vi "GetControlValues.vi"(11 "VI Name":string) -> (3 "Values":string[](array[string]))   [LabVIEW 2018, in "TracerLibrary.lvlib" / "Tracer.lvclass"]
uses:
  Tracer.lvclass
  Tracer_ClassAttributes.vi
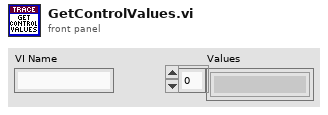
[diagram p1: front panel]
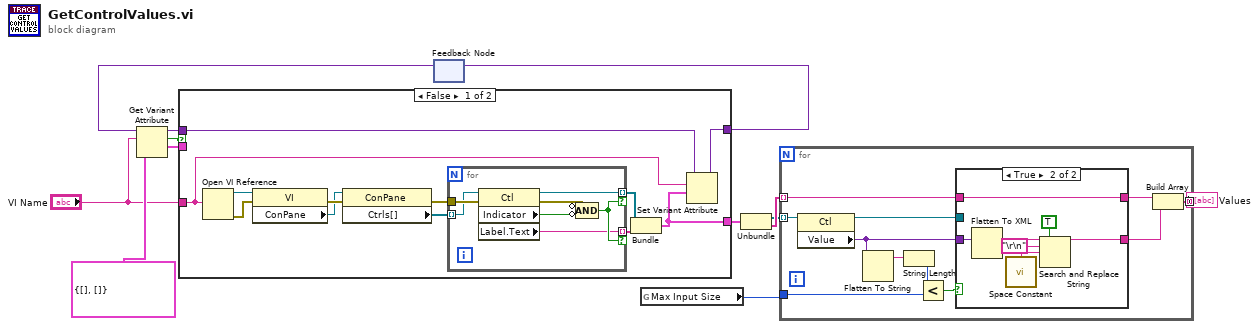
[diagram p0: block diagram]
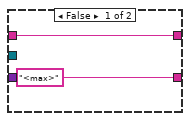
[diagram p2: hidden frame]
diagram:
  n1 = feedback #1() -> (w12:variant)  [unwired: 1 in]
  n2 = Get Variant Attribute(Variant=w12, name="VI Name", default value (empty Variant)=cluster{refnum<vi>[], string[]} {[], []} ("output cluster")) -> (duplicate Variant=w3:variant, found=w4:bool, value=w5:cluster{refnum<vi>[], string[]})  [unwired: 1 in, 1 out]
  n3 = case shown="False" w4 {
    tunnel: "VI Name" -> [w13 _]
    tunnel: w3 -> [w18 w32]
    tunnel: [w17 w32] -> w11
    tunnel: [w14 w33] -> w7
    tunnel: w5 -> [_ w33]
    frame False {
      n4 = Open VI Reference(vi path=w13) -> (vi reference=w21:refnum<vi>, error out=w23:errorcluster)  [unwired: 5 in]
      n5 = property class="VI"(reference=w21, error in=w23) -> (error out=w22:errorcluster, "ConPane"=w20:refnum<vi>)  [unwired: 1 out]
      n6 = property class="ConPane"(reference=w20, error in=w22) -> (error out=w24:errorcluster, "Ctrls[]"=w19:refnum<vi>[])  [unwired: 1 out]
      n7 = for {
        tunnel: w19 -> [w29] mode=indexing
        tunnel: [w28] -> w16 mode=indexing if=w27
        tunnel: w24 -> [w31]
        tunnel: [w25] -> w15 mode=indexing if=w27
        n8 = property class="Ctl"(reference=w29, error in=w31) -> (reference out=w28:refnum<vi>, error out=w30:errorcluster, "Indicator"=w26:bool, "Label.Text"=w25:string)
        n9 = Compound Arithmetic op=AND(invert w30, invert w26) -> (w27:bool)
      }
      n10 = Bundle(w16, w15) -> (w14:cluster{refnum<vi>[], string[]})  [unwired: 1 in]
      n11 = Set Variant Attribute(Variant=w18, name=w13, value=w14) -> (Variant out=w17:variant)  [unwired: 1 in, 2 out]
    }
    frame True {
    }
  }
  n12 = feedback-in #1(w11) -> ()
  n13 = global read "Tracer_ClassAttributes.vi" "Max Input Size"() -> (w1:i32)
  n14 = Unbundle(w7) -> (w8:refnum<vi>[], w9:string[])
  n15 = for {
    tunnel: w1 -> [w42]
    tunnel: w8 -> [w38] mode=indexing
    tunnel: w9 -> [w37] mode=indexing
    tunnel: [w34] -> w10 mode=concatenating
    n16 = property class="Ctl"(reference=w38) -> (reference out=w39:refnum<vi>, "Value"=w40:variant)  [unwired: 1 in, 1 out]
    n17 = Flatten To String(anything=w40) -> (data string=w44:string)  [unwired: 3 in, 2 out]
    n18 = String Length(string=w44) -> (length=w43:i32)
    n19 = Less?(x=w43, y=w42) -> (x < y?=w41:bool)
    n20 = case shown="True" w41 {
      tunnel: w40 -> [_ w53]
      tunnel: w39 -> [_ _]
      tunnel: w37 -> [w46 w52]
      tunnel: [w46 w52] -> w36
      tunnel: ["<max>" ("xml string") w50] -> w35
      frame False {
      }
      frame True {
        n21 = Flatten To XML(anything=w53) -> (xml string=w51:string)
        n22 = call <vilib>:"Space Constant.vi"() -> ("String"=w47:string)
        n23 = Search and Replace String(replace all?=TRUE ("replace all? (F)"), input string=w51, search string="\r\n", replace string=w47) -> (result string=w50:string)  [unwired: 4 in, 3 out]
      }
    }
    n24 = Build Array(w36, w35) -> (w34:string[])
  }
  "Values" <- w10
